vi "Auto Elevator.vi"(8 "High?":bool, 9 "Manual Speed":dbl, 10 "Elevator State":dbl, 11 "Elevator Mode":dbl) -> (3 "Finished?":bool)   [LabVIEW 2017]
uses:
  Common Code/Elevator Mode.ctl
  Common Code/Elevator State.ctl
  Robot Global Data.vi
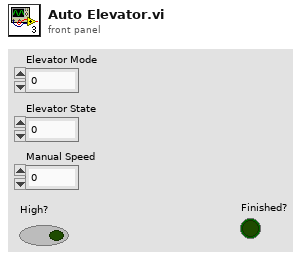
[diagram p1: front panel]
types:
  T1 = typedef "Elevator Mode.ctl" = enum16{"Semi Auto", "Manual", "Auto"}
  T2 = typedef "Elevator State.ctl" = enum16{"Idle", "Ground", "Mid", "Scale", "Switch"}
  T3 = typedef "Elevator Status Cluster.ctl" = cluster{"Finished":bool, "Elevator Power":dbl, "Elevator State":T2, "Elevator Mode":T1, "Elevator Height":dbl, "At Bottom?":bool, "At Top?":bool, "Scale high?":bool, "PID Output":dbl}
  T4 = typedef "Elevator Command Cluster.ctl" = cluster{"Elevator Mode":T1, "Elevator State":T2, "Manual Speed":dbl, "Reset Encoders":bool, "High?":bool, "Climb?":bool}
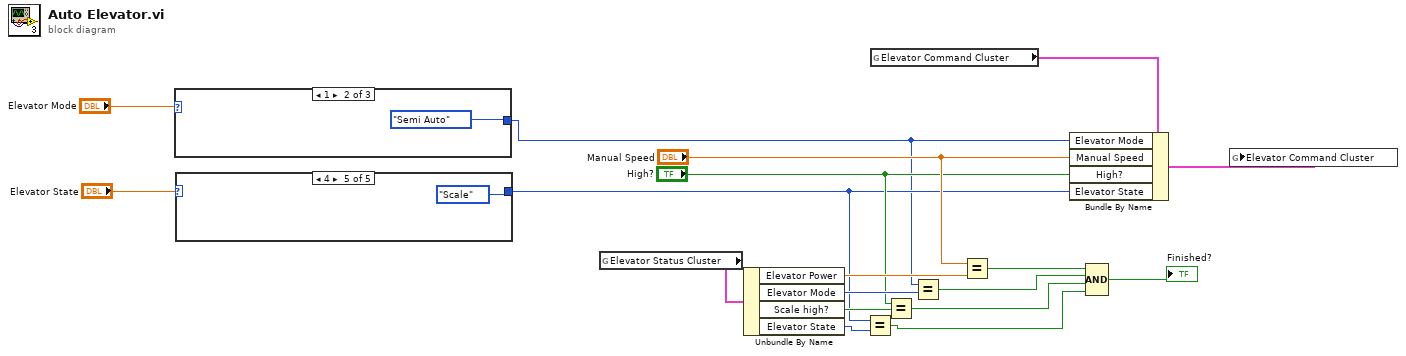
[diagram p0: block diagram]
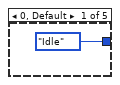
[diagram p2: hidden frame]
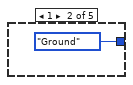
[diagram p3: hidden frame]
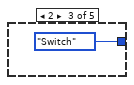
[diagram p4: hidden frame]
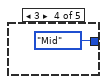
[diagram p5: hidden frame]
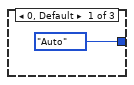
[diagram p6: hidden frame]
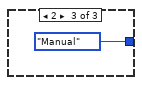
[diagram p7: hidden frame]
diagram:
  n1 = case shown="1" "Elevator Mode" {
    tunnel: [Elevator_Mode."Auto" ("Elevator Mode") Elevator_Mode."Semi Auto" ("Elevator Mode") Elevator_Mode."Manual" ("Elevator Mode")] -> w1
    frame 0, Default {
    }
    frame 1 {
    }
    frame 2 {
    }
  }
  n2 = case shown="4" "Elevator State" {
    tunnel: [Elevator_State."Idle" ("Elevator State") Elevator_State."Ground" ("Elevator State") Elevator_State."Switch" ("Elevator State") Elevator_State."Mid" ("Elevator State") Elevator_State."Scale" ("Elevator State")] -> w3
    frame 0, Default {
    }
    frame 1 {
    }
    frame 2 {
    }
    frame 3 {
    }
    frame 4 {
    }
  }
  n3 = global read "Robot Global Data.vi" "Elevator Status Cluster"() -> (w16:T3)
  n4 = Unbundle By Name(w16) -> ("Elevator Power"=w14:dbl, "Elevator Mode"=w12:T1, "Scale high?"=w10:bool, "Elevator State"=w4:T2)
  n5 = Equal?(x=w3, y=w4) -> (x = y?=w2:bool)
  n6 = global read "Robot Global Data.vi" "Elevator Command Cluster"() -> (w17:T4)
  n7 = Equal?(x="High?", y=w10) -> (x = y?=w8:bool)
  n8 = Equal?(x=w1, y=w12) -> (x = y?=w11:bool)
  n9 = Equal?(x="Manual Speed", y=w14) -> (x = y?=w13:bool)
  n10 = Bundle By Name(cluster=w17, "Elevator Mode"=w1, "Manual Speed"="Manual Speed", "High?"="High?", "Elevator State"=w3) -> (w18:T4)
  n11 = Compound Arithmetic op=AND(w13, w11, w8, w2) -> (→"Finished?":bool)
  n12 = global write "Robot Global Data.vi" "Elevator Command Cluster"(w18) -> ()
